vi "PH_gentec_M-Link.set Sets 2 change Flag.vi"(0 "i ref in":refnum<vi>, 5 "error in":errorcluster) -> (14 "i ref out":refnum<vi>, 19 "error out":errorcluster)   [LabVIEW 2014, in "PH_gentec_M-Link.lvlib"]
doc: "This VI indicates the wanted Settings at the GUI element."
uses:
  PH_gentec_M-Link.lvlib
  PH_Basics/PH_Powermeter_BaseClass/PH_Powermeter_BaseClass.State.ctl
  PH_Basics/PH_Powermeter_BaseClass/PH_Powermeter_BaseClass.lvlib
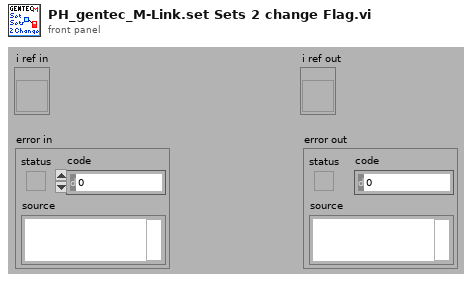
[diagram p1: front panel]
types:
  T1 = typedef "PH_Powermeter_BaseClass.lvlib/PH_Powermeter_BaseClass.i attribute.ctl" = cluster{"GUI References":T2, "Connection":T3, "Head Attributes":T5, "VISA resource":refnum<visa-resource-name>, "Energy":T6, "Service ID Energy":i32, "Wanted Settings":T7, "Current Settings":T7}
  T2 = typedef "PH_Powermeter_BaseClass.lvlib/PH_Powermeter_BaseClass.GUI Refs.ctl" = cluster{"Head Attributes":refnum<vi>, "Energy":refnum<vi>, "Connection":refnum<vi>, "VISA Resource":refnum<vi>, "Scaling Factor":refnum<vi>, "Range":refnum<vi>, "Wavelength":refnum<vi>, "Trigger Level":refnum<vi>, "Wanted Settings":refnum<vi>, "Current Settings":refnum<vi>}
  T3 = typedef "PH_Powermeter_BaseClass.lvlib/PH_Powermeter_BaseClass.Connection.ctl" = cluster{"failed checks":i8, "Timeout":bool, "Data read":string, "Failure":bool, "Error":bool, "State":T4}
  T4 = typedef "PH_Powermeter_BaseClass.lvlib/PH_Powermeter_BaseClass.State.ctl" = enum32{"off", "operating", "opened", "checked", "connected", "Sets to change", "running"}
  T5 = typedef "PH_Powermeter_BaseClass.lvlib/PH_Powermeter_BaseClass.Head Attributes.ctl" = cluster{"Instrument Type":string, "Head Version":string, "Head Name":string, "Serial Number":string, "Firmware":string, "Sensor Type":string, "MinimumRange":u32, "Maximum Range":u32, "Min Wavelength":i32, "Max Wavelength":i32}
  T6 = typedef "PH_Powermeter_BaseClass.lvlib/PH_Powermeter_BaseClass.Energy.ctl" = cluster{"current Value":dbl, "unscaled":dbl, "Scaling Factor":dbl}
  T7 = typedef "PH_Powermeter_BaseClass.lvlib/PH_gentec_BaseClass.Head Settings.ctl" = cluster{"Trigger Level":dbl, "Wavelength":u32, "Range":u32}
  T8 = typedef "PH_gentec_M-Link.lvlib/PH_gentec_M-Link.i attribute.ctl" = cluster{"GUI References":cluster{"Wanted Head Settings":refnum<vi>, "Current Head Settings":refnum<vi>, "Set Auto Range":refnum<vi>, "Trigger Polarity":refnum<vi>, "Trigger Source":refnum<vi>, "Waveform Averages":refnum<vi>, "Continuous":refnum<vi>, "get one Value":refnum<vi>}, "Wanted Head Settings":T9, "Current Head Settings":T9}
  T9 = typedef "PH_gentec_M-Link.lvlib/PH_gentec_M-Link.Head Settings.ctl" = cluster{"Measurement Mode":T10, "Enable Anticipation":bool, "Set Auto Range":bool, "Block Signal":bool, "Set Head Attenuator":bool, "Enable SSE":bool, "Trigger Polarity":T11, "Trigger Source":T12, "Waveform Averages":T13, "Set Zero":i32, "Current":i32, "Start Data Flow":bool}
  T10 = typedef "gentec-M-Link - Driver.lvlib/gentec-M-Link.Measurement Mode.ctl" = u16
  T11 = typedef "gentec-M-Link - Driver.lvlib/gentec-M-Link.Trigger Polarity.ctl" = u16
  T12 = typedef "gentec-M-Link - Driver.lvlib/gentec-M-Link.Trigger Source.ctl" = u16
  T13 = typedef "gentec-M-Link - Driver.lvlib/gentec-M-Link.Waveform Averages.ctl" = u16
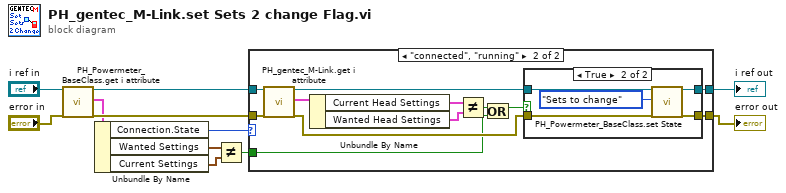
[diagram p0: block diagram]
diagram:
  n1 = call "PH_Powermeter_BaseClass.get i attribute.vi"("i ref in"="i ref in", "error in (no error)"="error in") -> ("i ref out"=w6:refnum<vi>, "i attribute"=w5:T1, "error out"=w8:errorcluster)  [unwired: 15 in]
  n2 = Unbundle By Name(w5) -> ("Connection.State"=w4:T4, "Wanted Settings"=w3:T7, "Current Settings"=w2:T7)
  n3 = Not Equal?(x=w3, y=w2) -> (x != y?=w1:bool)
  n4 = case shown="\"connected\", \"running\"" w4 {
    tunnel: [w12 w20] -> w11
    tunnel: [w13 w19] -> w10
    tunnel: w8 -> [w12 w18]
    tunnel: w6 -> [w13 w17]
    tunnel: w1 -> [_ w14]
    frame Default {
    }
    frame "connected", "running" {
      n5 = call "PH_gentec_M-Link.get i attribute.vi"("i ref in"=w17, "error in (no error)"=w18) -> ("i ref out"=w21:refnum<vi>, "i attribute"=w25:T8, "error out"=w22:errorcluster)  [unwired: 15 in]
      n6 = Unbundle By Name(w25) -> ("Current Head Settings"=w23:T9, "Wanted Head Settings"=w24:T9)
      n7 = Not Equal?(x=w23, y=w24) -> (x != y?=w16:bool)
      n8 = Or(x=w16, y=w14) -> (x .or. y?=w15:bool)
      n9 = case shown="True" w15 {
        tunnel: w22 -> [w26 w32]
        tunnel: w21 -> [w27 w31]
        tunnel: [w26 w30] -> w20
        tunnel: [w27 w29] -> w19
        frame False {
        }
        frame True {
          n10 = call "PH_Powermeter_BaseClass.set State.vi"("VI in"=w31, "State"=PH_Powermeter_BaseClass.State."Sets to change", "error in (no error)"=w32) -> ("VI out"=w29:refnum<vi>, "error out"=w30:errorcluster)  [unwired: 15 in]
        }
      }
    }
  }
  "error out" <- w11
  "i ref out" <- w10
